vi "DEMO.vi"() -> ()   [LabVIEW 2013]
panel:
  out "Output":string
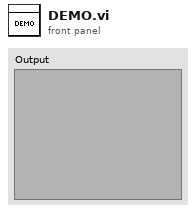
[diagram p1: front panel]
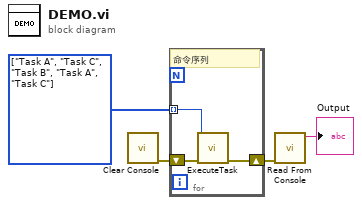
[diagram p0: block diagram]
diagram:
  w4 = enum16{"Task A", "Task B", "Task C"}[] [enum."Task A", enum."Task C", enum."Task B", enum."Task A", enum."Task C"] items=["Task A", "Task B", "Task C"]
  n1 = call "Clear Console.vi"() -> ("error out"=w3:errorcluster)  [unwired: 11 in]
  n2 = for {
    tunnel: w4 -> [w7] mode=indexing
    shift-right: [w5] -> w2
    shift-left: w3 -> [w6]
    # "命令序列"
    n3 = call "ExecuteTask.vi"("error in (no error)"=w6, "Task"=w7) -> ("error out"=w5:errorcluster)  [unwired: 9 in]
  }
  n4 = call "Read From Console.vi"("error in (no error)"=w2) -> ("Output"=→"Output":string)  [unwired: 9 in, 1 out]
